vi "test_multistream.vi"() -> ()   [LabVIEW 2023]
uses:
  <vilib>/picture/picture.llb/Draw True-Color Pixmap.vi
panel:
  out "pose (RF)":sgl[][](array[numeric])
  out "metadata (RF)":T1
  out "2D Picture (RF)":picture
  out "metadata (LF)":T1
  out "pose (LF)":sgl[][](array[numeric])
  out "2D Picture (LF)":picture
  in  "stop":bool
  in  "host":string="192.168.1.7"
  in  "path in":path=path "C:/Users/jcds/Documents/GitHub/hl2ss/extensions/client_labview/hl2ss_labview/hl2ss_ulm.dll"
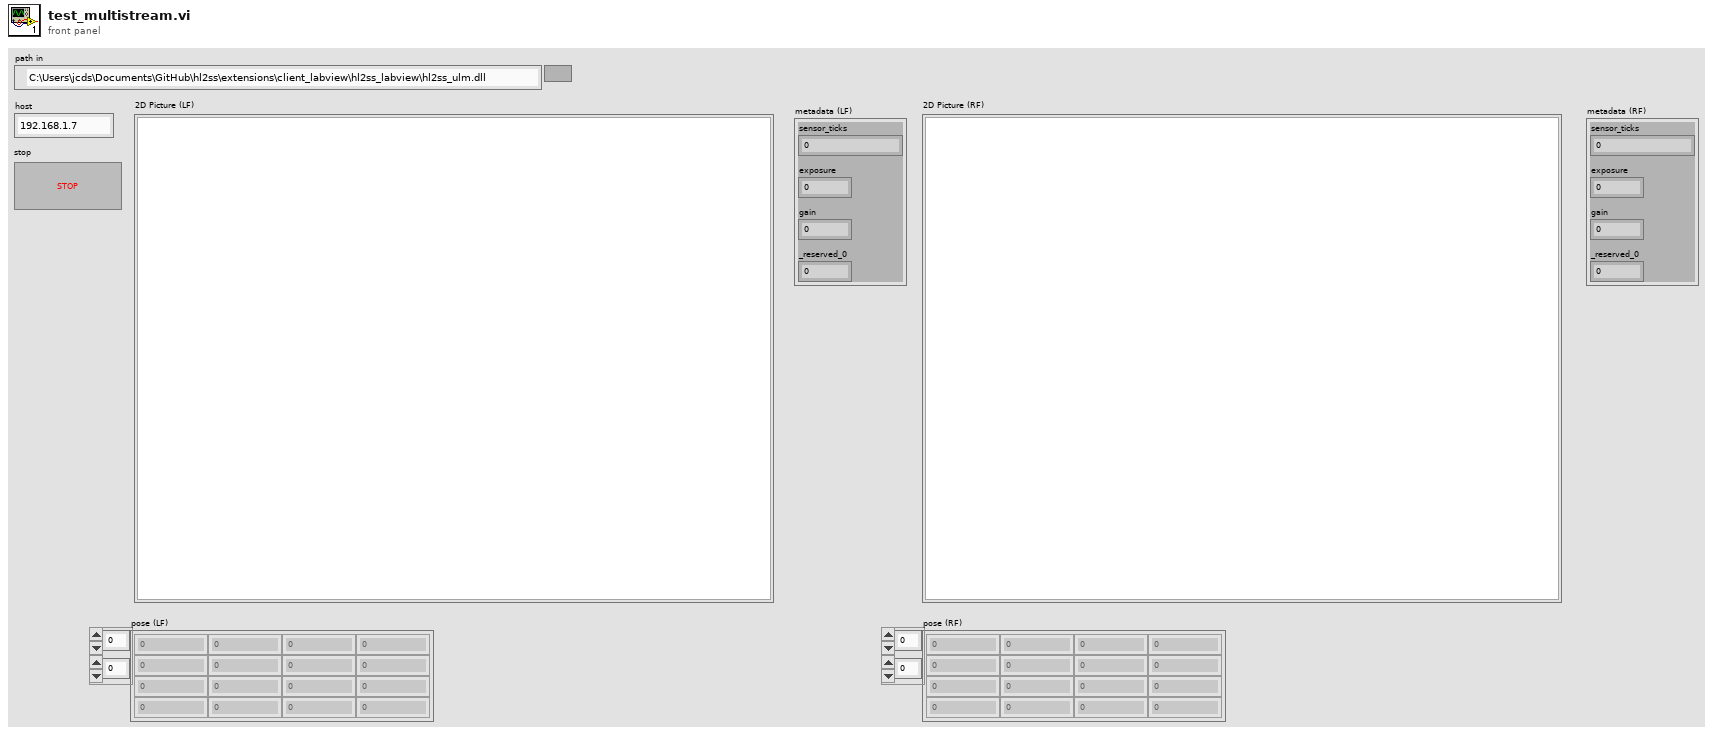
[diagram p1: front panel]
types:
  T1 = cluster{"sensor_ticks":u64, "exposure":u64, "gain":u32, "_reserved_0":u32}
  T2 = cluster{"chunk":u64, "mode":u8, "divisor":u8, "profile":u8, "level":u8, "bitrate":u32, "options_size":i64, "options_data":u64, "_reserved_0":u64}
  T3 = cluster{"frame_stamp":i64, "timestamp":u64, "payload_size":u32, "status":i32, "payload":u64, "pose":u64}
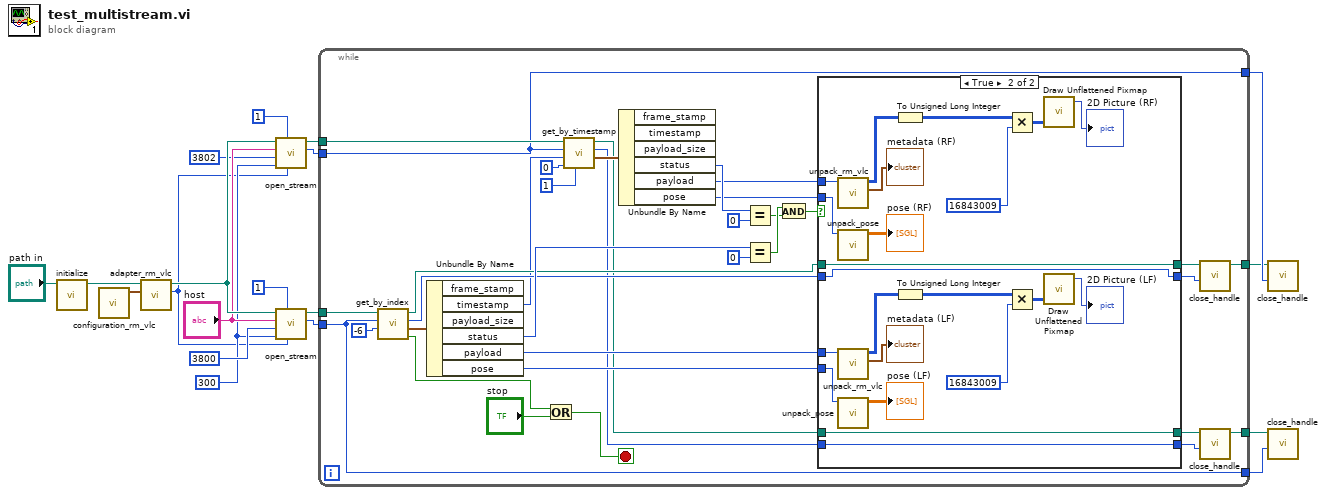
[diagram p0: block diagram]
diagram:
  w10 = u64 300 ("buffer_size")
  n1 = call "initialize.vi"("path in"="path in") -> ("path out"=w16:path)  [unwired: 9 in, 1 out]
  n2 = call "configuration_rm_vlc.vi"() -> ("configuration_rm_vlc"=w17:T2)  [unwired: 11 in]
  n3 = call "adapter_rm_vlc.vi"("configuration_rm_vlc"=w17, "path in"=w16) -> ("configuration"=w9:u64, "path out"=w14:path)  [unwired: 8 in]
  n4 = call "open_stream.vi"("configuration"=w9, "decoded"=u8 1, "buffer_size"=w10, "port"=u16 3802, "host"="host", "path in"=w14) -> ("handle"=w8:u64, "path out"=w7:path)  [unwired: 3 in, 1 out]
  n5 = call "open_stream.vi"("configuration"=w9, "decoded"=u8 1, "buffer_size"=w10, "port"=u16 3800, "host"="host", "path in"=w14) -> ("handle"=w15:u64, "path out"=w18:path)  [unwired: 3 in, 1 out]
  n6 = while {
    tunnel: w18 -> [w23]
    tunnel: [w42] -> w5
    tunnel: w15 -> [w24]
    tunnel: w8 -> [w25]
    tunnel: w7 -> [w39]
    tunnel: [w25] -> w6
    tunnel: [w24] -> w4
    tunnel: [w20] -> w3
    stop <- w47 stop-if-true
    n7 = call "get_by_index.vi"("frame_stamp"=i64 -6, "stream_handle"=w24, "path in"=w23) -> ("error"=w46:bool, "packet"=w52:T3, "packet_handle"=w48:u64, "path out"=w40:path)  [unwired: 5 in]
    n8 = Unbundle By Name(w52) -> ("timestamp"=w38:u64, "status"=w51:i32, "payload"=w43:u64, "pose"=w44:u64)  [unwired: 2 out]
    n9 = Or(x=w46, y="stop") -> (x .or. y?=w47:bool)
    n10 = call "get_by_timestamp.vi"("tiebreak_right"=1, "time_preference"=0, "timestamp"=w38, "stream_handle"=w25, "path in"=w39) -> ("packet"=w35:T3, "packet_handle"=w34:u64, "path out"=w33:path)  [unwired: 3 in, 1 out]
    n11 = Unbundle By Name(w35) -> ("status"=w31:i32, "payload"=w27:u64, "pose"=w26:u64)  [unwired: 3 out]
    n12 = Equal?(x=w31, y=0) -> (x = y?=w29:bool)
    n13 = Equal?(x=w51, y=0) -> (x = y?=w30:bool)
    n14 = And(x=w30, y=w29) -> (x .and. y?=w28:bool)
    n15 = case shown="True" w28 {
      tunnel: [w57 w79] -> w49
      tunnel: w48 -> [w57 w79]
      tunnel: w44 -> [_ w77]
      tunnel: w43 -> [_ w75]
      tunnel: w40 -> [w56 w78]
      tunnel: [w56 w78] -> w41
      tunnel: w34 -> [w54 w58]
      tunnel: w33 -> [w55 w59]
      tunnel: w27 -> [_ w62]
      tunnel: w26 -> [_ w61]
      tunnel: [w55 w59] -> w22
      tunnel: [w54 w58] -> w21
      frame False {
      }
      frame True {
        n16 = call "unpack_rm_vlc.vi"("payload"=w62) -> ("rm_vlc_metadata"=→"metadata (RF)":T1, "image"=w64:u8[][])  [unwired: 8 in, 1 out]
        n17 = call "unpack_pose.vi"("pose"=w61) -> ("pose"=→"pose (RF)":sgl[][])  [unwired: 9 in, 1 out]
        n18 = call "unpack_rm_vlc.vi"("payload"=w75) -> ("rm_vlc_metadata"=→"metadata (LF)":T1, "image"=w72:u8[][])  [unwired: 8 in, 1 out]
        n19 = call "unpack_pose.vi"("pose"=w77) -> ("pose"=→"pose (LF)":sgl[][])  [unwired: 9 in, 1 out]
        n20 = To Unsigned Long Integer(number=w64) -> (unsigned 32bit integer=w67:u32[][])
        n21 = To Unsigned Long Integer(number=w72) -> (unsigned 32bit integer=w71:u32[][])
        n22 = Multiply(x=w67, y=u32 16843009) -> (x*y=w65:u32[][])
        n23 = Multiply(x=w71, y=u32 16843009) -> (x*y=w69:u32[][])
        n24 = call-poly <vilib>:"Draw Unflattened Pixmap.vi"("data (RGB format)"=w65) -> ("new picture"=→"2D Picture (RF)":picture)  [unwired: 8 in]
        n25 = call-poly <vilib>:"Draw Unflattened Pixmap.vi"("data (RGB format)"=w69) -> ("new picture"=→"2D Picture (LF)":picture)  [unwired: 8 in]
      }
    }
    n26 = call "close_handle.vi"("handle"=w49, "path in"=w41) -> ("path out"=w42:path)  [unwired: 9 in]
    n27 = call "close_handle.vi"("handle"=w21, "path in"=w22) -> ("path out"=w20:path)  [unwired: 9 in]
  }
  n28 = call "close_handle.vi"("handle"=w6, "path in"=w5) -> ()  [unwired: 9 in, 1 out]
  n29 = call "close_handle.vi"("handle"=w4, "path in"=w3) -> ()  [unwired: 9 in, 1 out]
